vi "ex_CreatePacketHeader.vi"(0 "Attributes":T3[](array[typedef]) {"dX" format="%.2f"; "X0" format="%<%X\n%x>T"; "Timestamp" format="%<%X\n%x>T"; "Start Timestamp" format="%<%X\n%x>T"}, 1 "x_columns":u16(ring) items=["None", "One", "Multiple"], 2 "test":T1, 3 "UUT":T2, 5 "nChannels":i32, 7 "delimiter (Tab)":string="\t", 9 "special blocks":cluster{"one block's data":string[][]}[](array[cluster]), 11 "error in (no error)":errorcluster, 12 "Decimal Separator":string) -> (4 "spreadsheet string":string, 6 "string array":string[][](array[string]), 8 "X0 array":timestamp[](array[timestamp]) format="%<%X\n%x>T", 10 "dX array":dbl[](array[numeric]) format="%.2f", 13 "nPoints array":i32[](array[numeric]), 14 "max nPoints index":i32, 15 "error out":errorcluster)   [LabVIEW 2017]
uses:
  <vilib>/express/express shared/transition.llb/ex_WaveformAttribsPlus.ctl
  <vilib>/express/express output/ExFileWriteBlock.llb/ex_CheckAllT0DtEqualAttr.vi
panel:
  in  "dX format":string="%.;%g"
  in  "notes":string="X values guaranteed valid only for "
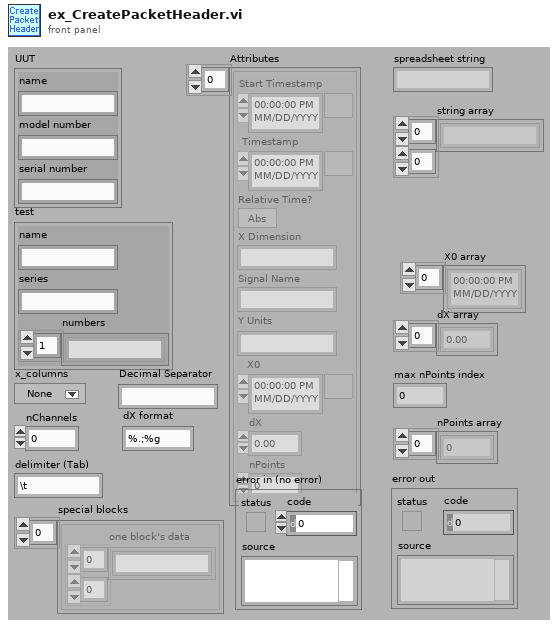
[diagram p1: front panel]
types:
  T1 = cluster{"name":string, "series":string, "numbers":string[]}
  T2 = cluster{"name":string, "model number":string, "serial number":string}
  T3 = typedef "ex_WaveformAttribsPlus.ctl" = cluster{"Start Timestamp":timestamp, "Timestamp":timestamp, "Relative Time?":bool, "X Dimension":string, "Signal Name":string, "Y Units":string, "X0":timestamp, "dX":dbl, "nPoints":i32}
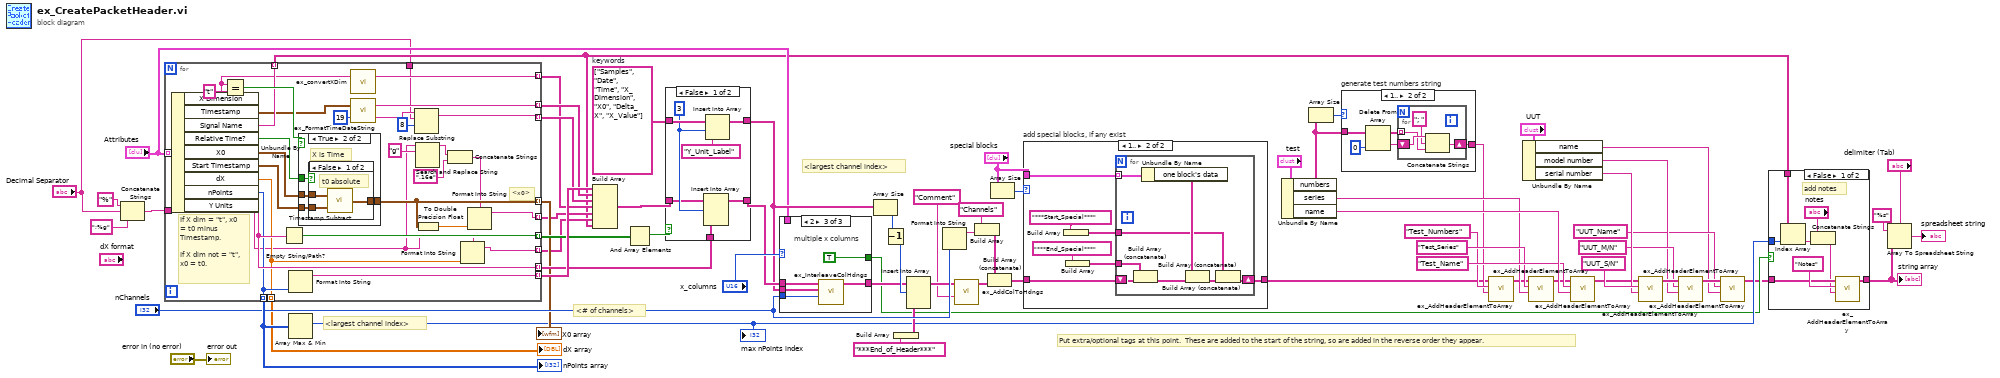
[diagram p0: block diagram]
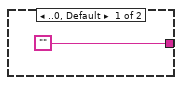
[diagram p2: hidden frame]
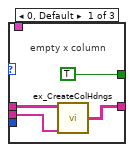
[diagram p5: hidden frame]
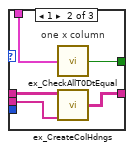
[diagram p6: hidden frame]
diagram:
  w58 = string[] ["Samples", "Date", "Time", "X_Dimension", "X0", "Delta_X", "X_Value"]  # keywords
  # "Put extra/optional tags at this point.  These are added to the start of the string, so are added in the reverse order they appear."
  # "<largest channel index>"
  # "<# of channels>"
  # "<largest channel index>"
  n1 = Concatenate Strings("%" ("string"), "Decimal Separator", ";%g" ("string")) -> (w2:string)
  n2 = for {
    tunnel: [w98] -> w50 mode=indexing
    tunnel: [w75] -> w51 mode=indexing
    tunnel: [w94] -> w32 mode=indexing
    tunnel: [w93] -> w45 mode=indexing
    tunnel: [w82] -> w46 mode=indexing
    tunnel: [w80] -> w47 mode=indexing
    tunnel: [w71] -> w48 mode=indexing
    tunnel: [w81] -> w49 mode=indexing
    tunnel: "Attributes" -> [w95] mode=indexing
    tunnel: [w85] -> w60 mode=indexing
    tunnel: [w86] -> w62 mode=indexing
    tunnel: [w88] -> w66 mode=indexing
    tunnel: [w84] -> w67 mode=indexing
    tunnel: w2 -> [w69]
    tunnel: "Decimal Separator" -> [w74]
    # "If X dim = \"t\", x0 = t0 minus Timestamp.\n\nIf X dim not = \"t\", x0 = t0."
    # "<x0>"
    n3 = Unbundle By Name(w95) -> ("X Dimension"=w89:string, "Timestamp"=w92:timestamp, "Signal Name"=w94:string, "Relative Time?"=w90:bool, "X0"=w87:timestamp, "Start Timestamp"=w83:timestamp, "dX"=w81:dbl, "nPoints"=w84:i32, "Y Units"=w86:string)
    n4 = Equal?(x=w89, y="t") -> (x = y?=w96:bool)
    n5 = Empty String/Path?(string/path=w86) -> (empty?=w85:bool)
    n6 = Format Into String(w84) -> (resulting string=w88:string)  [unwired: 3 in, 1 out]
    n7 = case shown="True" w96 {
      tunnel: [w99 w103] -> w71
      tunnel: w87 -> [w99 w101]
      tunnel: w90 -> [_ w102]
      tunnel: w83 -> [_ w100]
      frame False {
        # "X is NOT Time"
      }
      frame True {
        # "X is Time"
        n8 = case shown="False" w102 {
          tunnel: [w104 w107] -> w103
          tunnel: w101 -> [w106 w107]
          tunnel: w100 -> [w105 _]
          frame False {
            # "t0 absolute"
            n9 = call <vilib>:"Timestamp Subtract.vi"("y"=w105, "x"=w106) -> ("x - y"=w104:timestamp)
          }
          frame True {
            # "t0 relative"
          }
        }
      }
    }
    n10 = call <vilib>:"ex_convertXDim.vi"("x_dimension in"=w89) -> ("x_dimension out"=w93:string)  [unwired: 1 in, 1 out]
    n11 = call <vilib>:"ex_FormatTimeDateString.vi"("seconds precision (3)"=u32 19, "seconds since 1/1/1904"=w92) -> ("time string"=w76:string, "date string"=w98:string)
    n12 = Replace Substring(3:8 ("offset (0)"), 4:w74, 5:w76) -> (1:w75:string)  [unwired: 2 out]
    n13 = Search and Replace String(input string=w69, search string="g") -> (result string=w77:string)  [unwired: 1 in, 8 out]
    n14 = To Double Precision Float(number=w71) -> (double precision float=w72:dbl)
    n15 = Concatenate Strings(w77, ".16e" ("format")) -> (w70:string)
    n16 = Format Into String(format string=w69, w81) -> (resulting string=w80:string)  [unwired: 2 in, 1 out]
    n17 = Format Into String(format string=w70, w72) -> (resulting string=w82:string)  [unwired: 2 in, 1 out]
  }
  "nPoints array" <- w67
  "dX array" <- w49
  "X0 array" <- w48
  n18 = Array Max & Min(array=w67) -> (max index (indices)=w33:i32)  [unwired: 3 out]
  "max nPoints index" <- w33
  n19 = Build Array(w66, w50, w51, w45, w46, w47, w32) -> (w63:string[][])
  n20 = And Array Elements(Boolean array=w60) -> (logical AND=w61:bool)
  n21 = case shown="False" w61 {
    tunnel: w58 -> [w114 w116]
    tunnel: [w112 w116] -> w59
    tunnel: w63 -> [w110 w115]
    tunnel: w62 -> [w109 _]
    tunnel: [w108 w115] -> w64
    frame False {
      w111 = 3 ("index")
      n22 = Insert Into Array(array=w110, index (row)=w111, new element=w109) -> (w108:string[][])  [unwired: 1 in]
      n23 = Insert Into Array(array=w114, index=w111, new element="Y_Unit_Label" ("new element/subarray")) -> (w112:string[])
    }
    frame True {
    }
  }
  n24 = case shown="2" "x_columns" {
    tunnel: [w118 w123 w130] -> w55
    tunnel: w64 -> [w120 w125 w129]
    tunnel: w59 -> [w119 w124 w128]
    tunnel: "nChannels" -> [_ _ w127]
    tunnel: "Attributes" -> [_ w122 _]
    tunnel: [TRUE ("All dt and t0 equal?") w121 TRUE ("All dt and t0 equal?")] -> w31
    frame 0, Default {
      # "empty x column"
      n25 = call <vilib>:"ex_CreateColHdngs.vi"("col heading labels"=w119, "all col heading data"=w120) -> ("final col headings"=w118:string[][])  [unwired: 2 out]
    }
    frame 1 {
      # "one x column"
      n26 = call-poly <vilib>:"ex_CheckAllT0DtEqual.vi"("Attributes"=w122) -> ("All dt and t0 equal?"=w121:bool)
      n27 = call <vilib>:"ex_CreateColHdngs.vi"("col heading labels"=w124, "all col heading data"=w125) -> ("final col headings"=w123:string[][])  [unwired: 2 out]
    }
    frame 2 {
      # "multiple x columns"
      n28 = call <vilib>:"ex_InterleaveColHdngs.vi"("channels"=w127, "col heading tokens"=w128, "col heading data"=w129) -> ("modified heading data"=w130:string[][])  [unwired: 1 in, 5 out]
    }
  }
  n29 = Array Size(array=w59) -> (size(s)=w54:i32)
  n30 = Decrement(x=w54) -> (x-1=w57:i32)
  n31 = Build Array("***End_of_Header***") -> (w53:string[])
  n32 = Insert Into Array(array=w55, index (row)=w57, new element=w53) -> (w56:string[][])  [unwired: 1 in]
  n33 = Format Into String("nChannels") -> (resulting string=w39:string)  [unwired: 3 in, 1 out]
  n34 = call <vilib>:"ex_AddColToHdngs.vi"("new heading"="Comment", "headings"=w56) -> ("headings out"=w42:string[][])  [unwired: 5 out]
  n35 = Build Array("Channels" ("Channels"), w39) -> (w40:string[])
  n36 = Build Array (concatenate)(w40, w42) -> (w29:string[][])
  n37 = Array Size(array="special blocks") -> (size(s)=w28:i32)
  n38 = case "add special blocks, if any exist" shown="1.." w28 {
    tunnel: w29 -> [w131 w135]
    tunnel: "special blocks" -> [_ w138]
    tunnel: [w131 w134] -> w18
    frame ..0, Default {
    }
    frame 1.. {
      n39 = Build Array("***Start_Special***") -> (w133:string[])
      n40 = Build Array("***End_Special***") -> (w132:string[])
      n41 = for {
        tunnel: w138 -> [w145] mode=indexing
        tunnel: w133 -> [w140]
        tunnel: w132 -> [w139]
        shift-right: [w141] -> w134
        shift-left: w135 -> [w146]
        n42 = Build Array (concatenate)(w139, w146) -> (w144:string[][])
        n43 = Unbundle By Name(w145) -> ("one block's data"=w143:string[][])
        n44 = Build Array (concatenate)(w143, w144) -> (w142:string[][])
        n45 = Build Array (concatenate)(w140, w142) -> (w141:string[][])
      }
    }
  }
  n46 = Unbundle By Name("test") -> ("numbers"=w21:string[], "series"=w23:string, "name"=w26:string)
  n47 = Array Size(array=w21) -> (size(s)=w22:i32)
  n48 = case "generate test numbers string" shown="1.." w22 {
    tunnel: w21 -> [_ w152]
    tunnel: ["" w148] -> w19
    frame ..0, Default {
    }
    frame 1.. {
      n49 = Delete From Array(array=w152, index=0) -> (deleted portion=w150:string, array with subset deleted=w149:string[])  [unwired: 1 in]
      n50 = for {
        shift-right: [w153] -> w148
        shift-left: w150 -> [w156]
        tunnel: w149 -> [w155] mode=indexing
        n51 = Concatenate Strings(w156, "; ", w155) -> (w153:string)
      }
    }
  }
  n52 = call <vilib>:"ex_AddHeaderElementToArray.vi"("string"=w19, "name"="Test_Numbers", "string array in"=w18) -> ("string array out"=w17:string[][])  [unwired: 1 in, 7 out]
  n53 = Unbundle By Name("UUT") -> ("name"=w6:string, "model number"=w8:string, "serial number"=w13:string)
  n54 = call <vilib>:"ex_AddHeaderElementToArray.vi"("string"=w23, "name"="Test_Series", "string array in"=w17) -> ("string array out"=w16:string[][])  [unwired: 1 in, 7 out]
  n55 = call <vilib>:"ex_AddHeaderElementToArray.vi"("string"=w26, "name"="Test_Name", "string array in"=w16) -> ("string array out"=w12:string[][])  [unwired: 1 in, 7 out]
  n56 = call <vilib>:"ex_AddHeaderElementToArray.vi"("string"=w13, "name"="UUT_S/N", "string array in"=w12) -> ("string array out"=w11:string[][])  [unwired: 1 in, 7 out]
  n57 = call <vilib>:"ex_AddHeaderElementToArray.vi"("string"=w8, "name"="UUT_M/N", "string array in"=w11) -> ("string array out"=w10:string[][])  [unwired: 1 in, 7 out]
  n58 = call <vilib>:"ex_AddHeaderElementToArray.vi"("string"=w6, "name"="UUT_Name", "string array in"=w10) -> ("string array out"=w5:string[][])  [unwired: 1 in, 7 out]
  n59 = case shown="False" w31 {
    tunnel: w5 -> [w158 w165]
    tunnel: [w159 w165] -> w38
    tunnel: w33 -> [w162 _]
    tunnel: w32 -> [w161 _]
    frame False {
      # "add notes"
      n60 = Index Array(array=w161, index=w162) -> (element=w163:string)
      n61 = Concatenate Strings("notes", w163) -> (w157:string)
      n62 = call <vilib>:"ex_AddHeaderElementToArray.vi"("string"=w157, "name"="Notes" ("Notes"), "string array in"=w158) -> ("string array out"=w159:string[][])  [unwired: 1 in, 7 out]
    }
    frame True {
    }
  }
  "string array" <- w38
  n63 = Array To Spreadsheet String(delimiter (Tab)="delimiter (Tab)", array=w38, 3:"%s" ("format string")) -> (spreadsheet string=→"spreadsheet string":string)
  "error out" <- "error in (no error)"
